vi "Thread.Set Runnable.vi"(10 "Runnable":refnum<class "Runnable.lvclass">, 11 "Thread in":refnum<class "Thread.lvclass">) -> (3 "Thread out":refnum<class "Thread.lvclass">)   [LabVIEW 2017, in "Thread.lvclass"]
uses:
  Thread.lvclass
  Runnable.lvclass
  Thread.lvclass/Thread.ctl
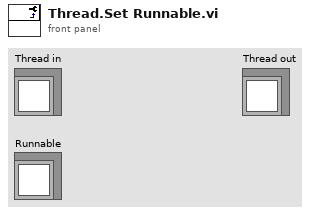
[diagram p1: front panel]
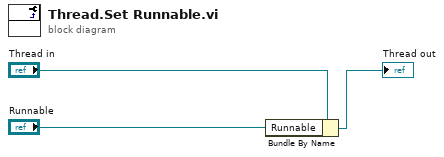
[diagram p0: block diagram]
diagram:
  n1 = Bundle By Name(cluster="Thread in", "Runnable"="Runnable") -> (→"Thread out":refnum<class "Thread.lvclass">)
